vi "timeStampToString.vi"(1 "Time Stamp":timestamp) -> (0 "Time Stamp String":string)   [LabVIEW 2017, in "Error Log.lvlib" / "Record.lvclass"]
uses:
  Record.lvclass
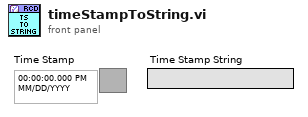
[diagram p1: front panel]
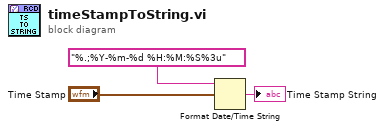
[diagram p0: block diagram]
diagram:
  n1 = Format Date/Time String(time format string (%c)="%.;%Y-%m-%d %H:%M:%S%3u", seconds (now)="Time Stamp") -> (date/time string=→"Time Stamp String":string)  [unwired: 1 in]
